vi "AutoDriveChooseState.vi"(8 "error in (no error)":errorcluster, 11 "AutoMode":T2) -> (0 "error out":errorcluster, 3 "Current State":T1)   [LabVIEW 2013]
doc: "Choose the next state from Drive, based upon the AutoMode (One / Two ball, front / in collector)."
uses:
  AutoMode.ctl
  AutoStates.ctl
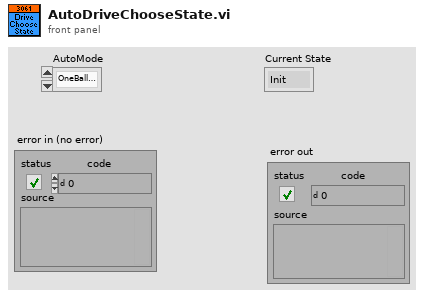
[diagram p1: front panel]
types:
  T1 = typedef "AutoStates.ctl" = enum16{"Init", "LowerArmCheckGoal", "DriveBack", "Collect", "StopCollect", "LiftArm", "RaiseServo", "Drive", "ShootCollectorUp", "RaiseArm", "ShootCollectorDown", "Rotate1", "Rotate2***", "Stop"}
  T2 = typedef "AutoMode.ctl" = enum16{"OneBallFront", "OneBallCollector", "TwoBallNormal", "TwoBallHot"}
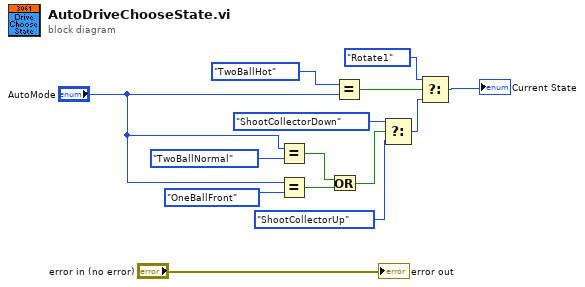
[diagram p0: block diagram]
diagram:
  n1 = Equal?(x="AutoMode", y=AutoMode."TwoBallNormal") -> (x = y?=w3:bool)
  n2 = Equal?(x="AutoMode", y=AutoMode."OneBallFront") -> (x = y?=w4:bool)
  n3 = Or(x=w3, y=w4) -> (x .or. y?=w8:bool)
  n4 = Equal?(x=AutoMode."TwoBallHot" ("y"), y="AutoMode") -> (x = y?=w12:bool)
  n5 = Select(t=AutoStates."ShootCollectorDown" ("Enum"), s=w8, f=AutoStates."ShootCollectorUp") -> (s? t:f=w9:T1)
  n6 = Select(t=AutoStates."Rotate1" ("Enum"), s=w12, f=w9) -> (s? t:f=→"Current State":T1)
  "error out" <- "error in (no error)"
